vi "模拟138译码器.vi"() -> ()   [LabVIEW 2012, in "触发器.lvlib"]
panel:
  out "Y7":bool
  out "Y6":bool
  out "Y5":bool
  out "Y4":bool
  out "Y3":bool
  out "Y2":bool
  out "Y1":bool
  out "Y0":bool
  in  "A2":bool
  in  "A1":bool
  in  "A0":bool
  in  "S3":bool
  in  "S2":bool
  in  "S1":bool
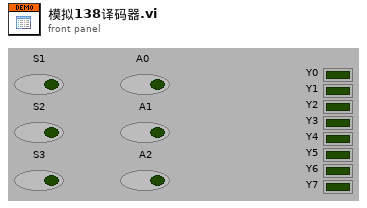
[diagram p1: front panel]
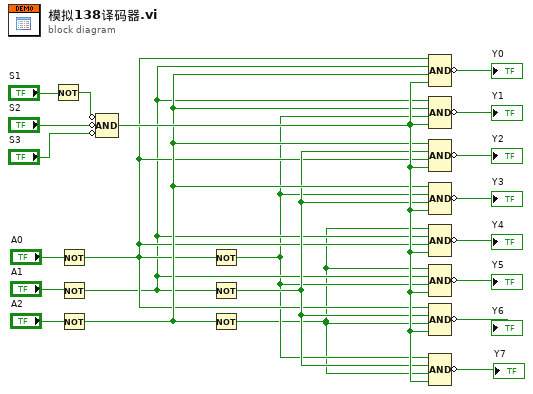
[diagram p0: block diagram]
diagram:
  n1 = Not(x="S1") -> (.not. x?=w21:bool)
  n2 = Not(x="A0") -> (.not. x?=w4:bool)
  n3 = Not(x="A1") -> (.not. x?=w3:bool)
  n4 = Not(x="A2") -> (.not. x?=w6:bool)
  n5 = Compound Arithmetic op=AND(invert w21, invert "S2", invert "S3") -> (w14:bool)
  n6 = Not(x=w4) -> (.not. x?=w2:bool)
  n7 = Not(x=w3) -> (.not. x?=w5:bool)
  n8 = Not(x=w6) -> (.not. x?=w1:bool)
  n9 = Compound Arithmetic op=AND(w4, w3, w6, w14) -> (invert →"Y0":bool)
  n10 = Compound Arithmetic op=AND(w3, w6, w2, w14) -> (invert →"Y1":bool)
  n11 = Compound Arithmetic op=AND(w6, w5, w4, w14) -> (invert →"Y2":bool)
  n12 = Compound Arithmetic op=AND(w6, w2, w5, w14) -> (invert →"Y3":bool)
  n13 = Compound Arithmetic op=AND(w1, w3, w4, w14) -> (invert →"Y4":bool)
  n14 = Compound Arithmetic op=AND(w1, w3, w2, w14) -> (invert →"Y5":bool)
  n15 = Compound Arithmetic op=AND(w4, w5, w1, w14) -> (invert →"Y6":bool)
  n16 = Compound Arithmetic op=AND(w2, w5, w1, w14) -> (invert →"Y7":bool)
